vi "GlobalWhatAroundMe.vi"() -> ()   [LabVIEW 2010]
panel:
  out "WhatAroundMe?":cluster{"T":dbl, "Range":dbl, "Bearing":dbl}[](array[cluster])
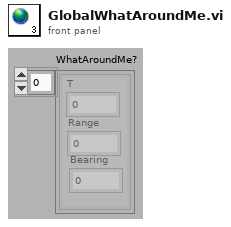
[diagram p1: front panel]
diagram:
